vi "GetCellInfo.vi"() -> ()   [LabVIEW 2013]
uses:
  XML/Public XML/RowDataFilter.ctl
  XML.lvlib
panel:
  in  "Node Text Value":string
  in  "Rows 3":string[](array[string])=["<table:table-row xmlns:table=\"urn:oasis:names:tc:opendocument:xmlns:table:1.0\" table:style-name=\"ro1\"><table:table-cell xmlns:calcext=\"urn:org:documentfoundation:names:experimental:calc:xmlns:calcext:1.0\" calcext:value-type=\"string\" xmlns:office=\"urn:oasis:names:tc:opendocument:xmlns:office:1.0\" office:value-type=\"string\"><text:p xmlns:text=\"urn:oasis:names:tc:opendocument:xmlns:text:1.0\">Title1</text:p></table:table-cell><table:table-cell table:number-columns-repeated=\"12\"/></table:table-row>", "<table:table-row xmlns:table=\"urn:oasis:names:tc:opendocument:xmlns:table:1.0\" table:style-name=\"ro2\"><table:table-cell/><table:table-cell xmlns:calcext=\"urn:org:documentfoundation:names:experimental:calc:xmlns:calcext:1.0\" calcext:value-type=\"string\" xmlns:office=\"urn:oasis:names:tc:opendocument:xmlns:office:1.0\" office:value-type=\"string\"><text:p xmlns:text=\"urn:oasis:names:tc:opendocument:xmlns:text:1.0\">aaaaaaaaaaaaaaaaaaaaa</text:p></table:table-cell><table:table-cell table:number-columns-repeated=\"5\"/><table:table-cell xmlns:calcext=\"urn:org:documentfoundation:names:experimental:calc:xmlns:calcext:1.0\" calcext:value-type=\"string\" xmlns:office=\"urn:oasis:names:tc:opendocument:xmlns:office:1.0\" office:value-type=\"string\"><text:p xmlns:text=\"urn:oasis:names:tc:opendocument:xmlns:text:1.0\">H2</text:p></table:table-cell><table:table-cell table:number-columns-repeated=\"5\"/></table:table-row>", "<table:table-row xmlns:table=\"urn:oasis:names:tc:opendocument:xmlns:table:1.0\" table:style-name=\"ro2\"><table:table-cell/><table:table-cell xmlns:calcext=\"urn:org:documentfoundation:names:experimental:calc:xmlns:calcext:1.0\" calcext:value-type=\"string\" xmlns:office=\"urn:oasis:names:tc:opendocument:xmlns:office:1.0\" office:value-type=\"string\"><text:p xmlns:text=\"urn:oasis:names:tc:opendocument:xmlns:text:1.0\">bbbbbbbbbbbbbbbbbbbbb</text:p></table:table-cell><table:table-cell table:number-columns-repeated=\"11\"/></table:table-row>", "<table:table-row xmlns:table=\"urn:oasis:names:tc:opendocument:xmlns:table:1.0\" table:style-name=\"ro2\"><table:table-cell/><table:table-cell xmlns:calcext=\"urn:org:documentfoundation:names:experimental:calc:xmlns:calcext:1.0\" calcext:value-type=\"string\" xmlns:office=\"urn:oasis:names:tc:opendocument:xmlns:office:1.0\" office:value-type=\"string\"><text:p xmlns:text=\"urn:oasis:names:tc:opendocument:xmlns:text:1.0\">ccccccccccccccccccccc</text:p></table:table-cell><table:table-cell table:number-columns-repeated=\"11\"/></table:table-row>", "<table:table-row xmlns:table=\"urn:oasis:names:tc:opendocument:xmlns:table:1.0\" table:style-name=\"ro2\"><table:table-cell/><table:table-cell xmlns:calcext=\"urn:org:documentfoundation:names:experimental:calc:xmlns:calcext:1.0\" calcext:value-type=\"string\" xmlns:office=\"urn:oasis:names:tc:opendocument:xmlns:office:1.0\" office:value-type=\"string\"><text:p xmlns:text=\"urn:oasis:names:tc:opendocument:xmlns:text:1.0\">ddddddddddddddddddddd</text:p></table:table-cell><table:table-cell table:number-columns-repeated=\"11\"/></table:table-row>", "<table:table-row xmlns:table=\"urn:oasis:names:tc:opendocument:xmlns:table:1.0\" table:style-name=\"ro1\"><table:table-cell xmlns:calcext=\"urn:org:documentfoundation:names:experimental:calc:xmlns:calcext:1.0\" calcext:value-type=\"string\" xmlns:office=\"urn:oasis:names:tc:opendocument:xmlns:office:1.0\" office:value-type=\"string\"><text:p xmlns:text=\"urn:oasis:names:tc:opendocument:xmlns:text:1.0\">Title2</text:p></table:table-cell><table:table-cell table:number-columns-repeated=\"12\"/></table:table-row>", "<table:table-row xmlns:table=\"urn:oasis:names:tc:opendocument:xmlns:table:1.0\" table:style-name=\"ro2\"><table:table-cell/><table:table-cell xmlns:calcext=\"urn:org:documentfoundation:names:experimental:calc:xmlns:calcext:1.0\" calcext:value-type=\"string\" xmlns:office=\"urn:oasis:names:tc:opendocument:xmlns:office:1.0\" office:value-type=\"string\"><text:p xmlns:text=\"urn:oasis:names:tc:opendocument:xmlns:text:1.0\">eeeeeeeeeeeeeeeeeeeee</text:p></table:table-cell><table:table-cell table:number-columns-repeated=\"11\"/></table:table-row>", "<table:table-row xmlns:table=\"urn:oasis:names:tc:opendocument:xmlns:table:1.0\" table:style-name=\"ro2\"><table:table-cell/><table:table-cell xmlns:calcext=\"urn:org:documentfoundation:names:experimental:calc:xmlns:calcext:1.0\" calcext:value-type=\"string\" xmlns:office=\"urn:oasis:names:tc:opendocument:xmlns:office:1.0\" office:value-type=\"string\"><text:p xmlns:text=\"urn:oasis:names:tc:opendocument:xmlns:text:1.0\">ffffffffffffffffffffffffffffffffffffffff</text:p></table:table-cell><table:table-cell table:number-columns-repeated=\"11\"/></table:table-row>", "<table:table-row xmlns:table=\"urn:oasis:names:tc:opendocument:xmlns:table:1.0\" table:style-name=\"ro1\"><table:table-cell/><table:table-cell xmlns:calcext=\"urn:org:documentfoundation:names:experimental:calc:xmlns:calcext:1.0\" calcext:value-type=\"string\" xmlns:office=\"urn:oasis:names:tc:opendocument:xmlns:office:1.0\" office:value-type=\"string\"><text:p xmlns:text=\"urn:oasis:names:tc:opendocument:xmlns:text:1.0\">ggggggggggggggggggggg</text:p></table:table-cell><table:table-cell table:number-columns-repeated=\"11\"/></table:table-row>", "<table:table-row xmlns:table=\"urn:oasis:names:tc:opendocument:xmlns:table:1.0\" table:number-rows-repeated=\"5\" table:style-name=\"ro1\"><table:table-cell table:number-columns-repeated=\"13\"/></table:table-row>", "<table:table-row xmlns:table=\"urn:oasis:names:tc:opendocument:xmlns:table:1.0\" table:style-name=\"ro1\"><table:table-cell table:number-columns-repeated=\"4\"/><table:table-cell xmlns:calcext=\"urn:org:documentfoundation:names:experimental:calc:xmlns:calcext:1.0\" calcext:value-type=\"string\" xmlns:office=\"urn:oasis:names:tc:opendocument:xmlns:office:1.0\" office:value-type=\"string\"><text:p xmlns:text=\"urn:oasis:names:tc:opendocument:xmlns:text:1.0\">E16</text:p></table:table-cell><table:table-cell table:number-columns-repeated=\"8\"/></table:table-row>", "<table:table-row xmlns:table=\"urn:oasis:names:tc:opendocument:xmlns:table:1.0\" table:number-rows-repeated=\"10\" table:style-name=\"ro1\"><table:table-cell table:number-columns-repeated=\"13\"/></table:table-row>", "<table:table-row xmlns:table=\"urn:oasis:names:tc:opendocument:xmlns:table:1.0\" table:style-name=\"ro1\"><table:table-cell table:number-columns-repeated=\"12\"/><table:table-cell xmlns:calcext=\"urn:org:documentfoundation:names:experimental:calc:xmlns:calcext:1.0\" calcext:value-type=\"string\" xmlns:office=\"urn:oasis:names:tc:opendocument:xmlns:office:1.0\" office:value-type=\"string\"><text:p xmlns:text=\"urn:oasis:names:tc:opendocument:xmlns:text:1.0\">M26</text:p></table:table-cell></table:table-row>"]
  out "Cell Info":string[][](array[string])
  out "Table Data":string[][](array[string])
  in  "Rows 2":string[](array[string])
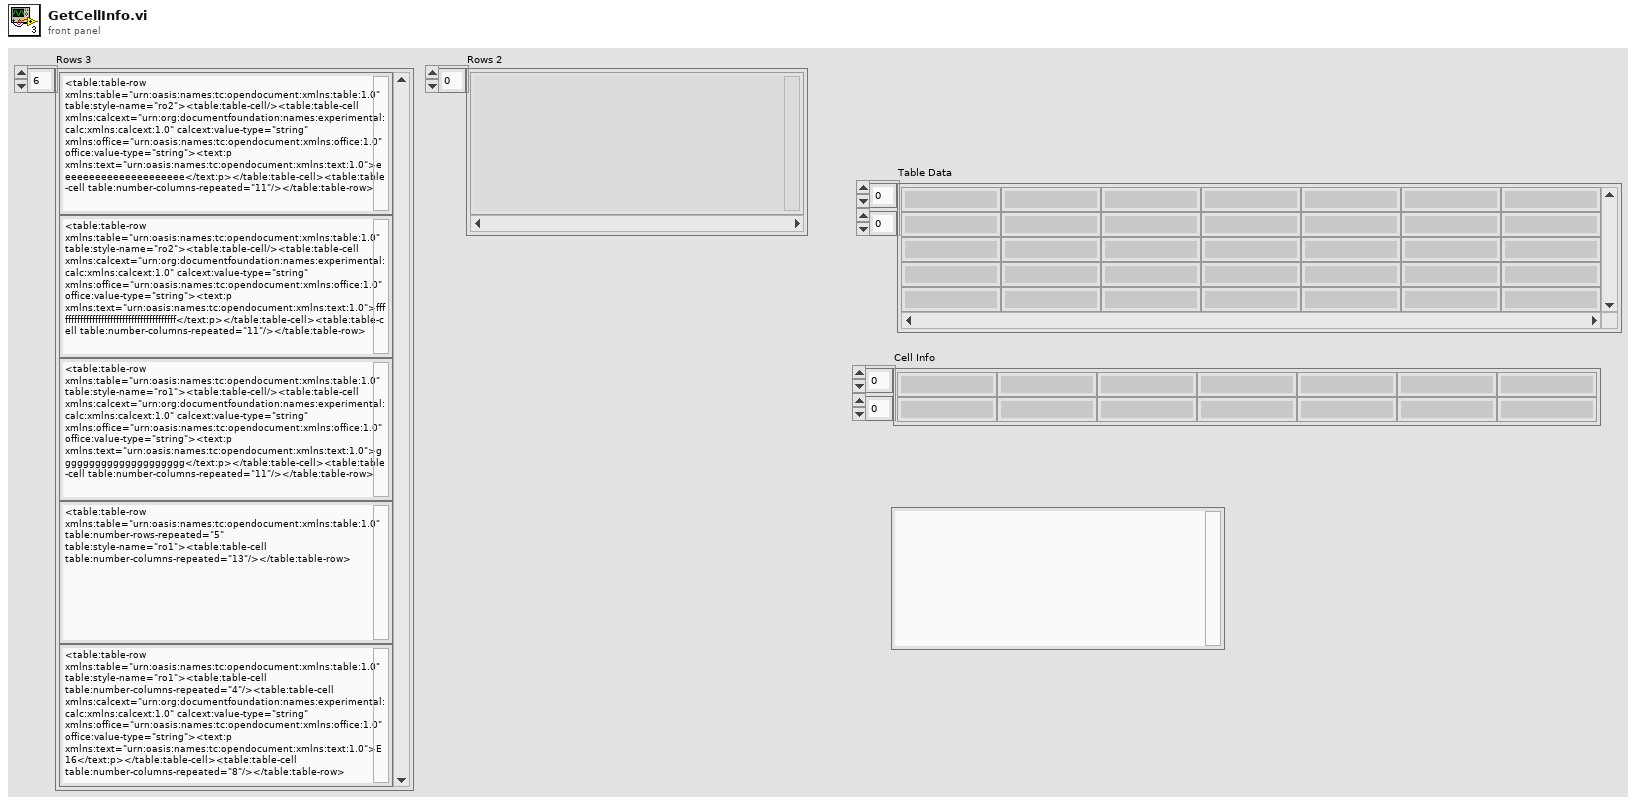
[diagram p1: front panel]
types:
  T1 = typedef "RowDataFilter.ctl" = enum16{"No Filter - Error", "Row Values", "Row Data", "#Rows Repeated", "#Columns Repeated"}
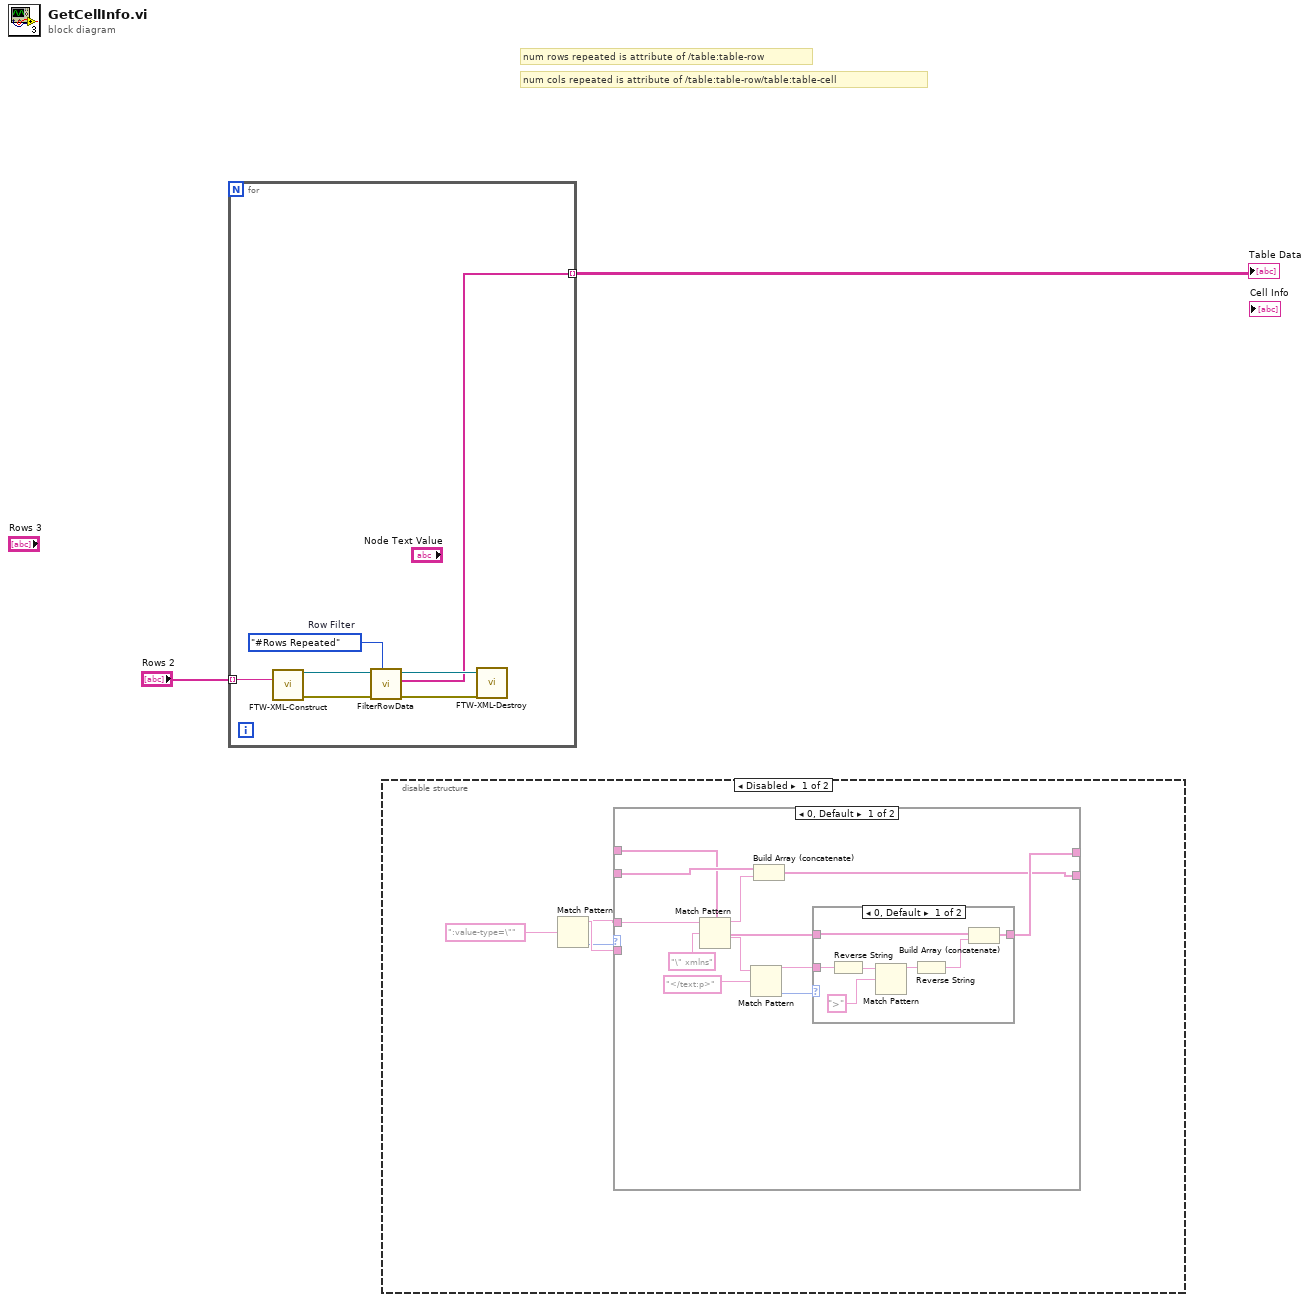
[diagram p0: block diagram]
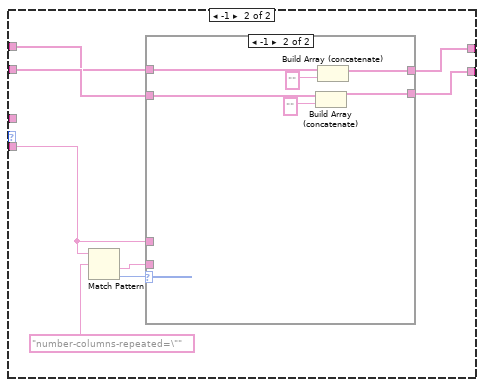
[diagram p3: hidden frame]
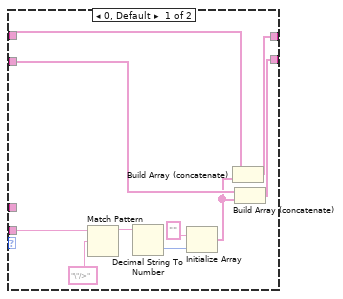
[diagram p4: hidden frame]
diagram:
  # "num cols repeated is attribute of /table:table-row/table:table-cell"
  # "num rows repeated is attribute of /table:table-row"
  n1 = for {
    tunnel: "Rows 2" -> [w9] mode=indexing
    tunnel: [w4] -> w1 mode=indexing
    w8 = RowDataFilter."#Rows Repeated"  # Row Filter
    n2 = call "FTW-XML-Construct.vi"("XML String"=w9) -> ("XML Document"=w5:refnum<k20>, "error out"=w3:errorcluster)  [unwired: 13 in]
    n3 = call "FilterRowData.vi"("Row Filter"=w8, "error in (no error)"=w3, "Row XML Node"=w5) -> ("error out"=w6:errorcluster, "Row Data"=w4:string[], "XML Node Out"=w7:refnum<k20>)  [unwired: 2 in, 1 out]
    n4 = call "FTW-XML-Destroy.vi"("XML Node"=w7, "error in"=w6) -> ()  [unwired: 13 in, 1 out]
  }
  "Table Data" <- w1
  n5 = disable-structure shown="Disabled" {
    frame Disabled {
      n6 = Match Pattern(regular expression=":value-type=\"") -> (string=w12:string, before substring=w10:string, offset past match=w11:i32)  [unwired: 1 in, 2 out]
      n7 = case shown="0, Default" w11 {
        tunnel: _ -> [w22 w37]
        tunnel: [w14 w34] -> _
        tunnel: w10 -> [w24 _]
        tunnel: _ -> [w17 w36]
        tunnel: [w15 w35] -> _
        tunnel: w12 -> [_ w33]
        frame 0, Default {
          n8 = Match Pattern(string=w24, regular expression="\" xmlns") -> (before substring=w21:string, after substring=w16:string)  [unwired: 1 in, 2 out]
          n9 = Match Pattern(string=w16, regular expression="</text:p>") -> (before substring=w19:string, offset past match=w18:i32)  [unwired: 1 in, 2 out]
          n10 = Build Array (concatenate)(w22, w21) -> (w14:string[])
          n11 = case shown="0, Default" w18 {
            tunnel: w19 -> [w31 _]
            tunnel: w17 -> [w27 w32]
            tunnel: [w25 w32] -> w15
            frame 0, Default {
              n12 = Reverse String(1:w31) -> (0:w30:string)
              n13 = Match Pattern(string=w30, regular expression=">") -> (before substring=w28:string)  [unwired: 1 in, 3 out]
              n14 = Reverse String(1:w28) -> (0:w26:string)
              n15 = Build Array (concatenate)(w27, w26) -> (w25:string[])
            }
            frame -1 {
            }
          }
        }
        frame -1 {
          n16 = Match Pattern(string=w33, regular expression="number-columns-repeated=\"") -> (after substring=w39:string, offset past match=w38:i32)  [unwired: 1 in, 2 out]
          n17 = case shown="-1" w38 {
            tunnel: w39 -> [w50 _]
            tunnel: w36 -> [w45 w54]
            tunnel: [w44 w53] -> w35
            tunnel: w37 -> [w43 w51]
            tunnel: [w41 w52] -> w34
            tunnel: w33 -> [_ _]
            frame 0, Default {
              n18 = Match Pattern(string=w50, regular expression="\"/>") -> (before substring=w48:string)  [unwired: 1 in, 3 out]
              n19 = Decimal String To Number(string=w48) -> (number=w47:i32)  [unwired: 2 in, 1 out]
              n20 = Initialize Array("", w47) -> (w42:string[])
              n21 = Build Array (concatenate)(w45, w42) -> (w44:string[])
              n22 = Build Array (concatenate)(w43, w42) -> (w41:string[])
            }
            frame -1 {
              n23 = Build Array (concatenate)(w51, "") -> (w52:string[])
              n24 = Build Array (concatenate)(w54, "") -> (w53:string[])
            }
          }
        }
      }
    }
    frame Enabled {
    }
  }
